vi "DecodeSymbols.vi"(10 "InputValid":bool, 11 "Symbol":T1=enum."Marker") -> (2 "Output Valid":bool, 3 "WWVB":u64 format="%.0x")   [LabVIEW 2019]
uses:
  TypeDefs/TimeSymbol.ctl
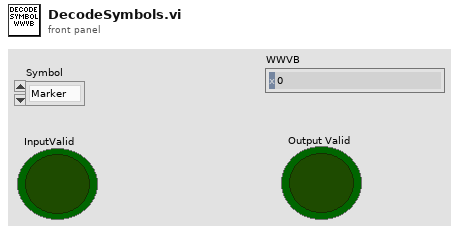
[diagram p1: front panel]
types:
  T1 = typedef "TimeSymbol.ctl" = enum16{"0", "1", "Marker", "Invalid"}
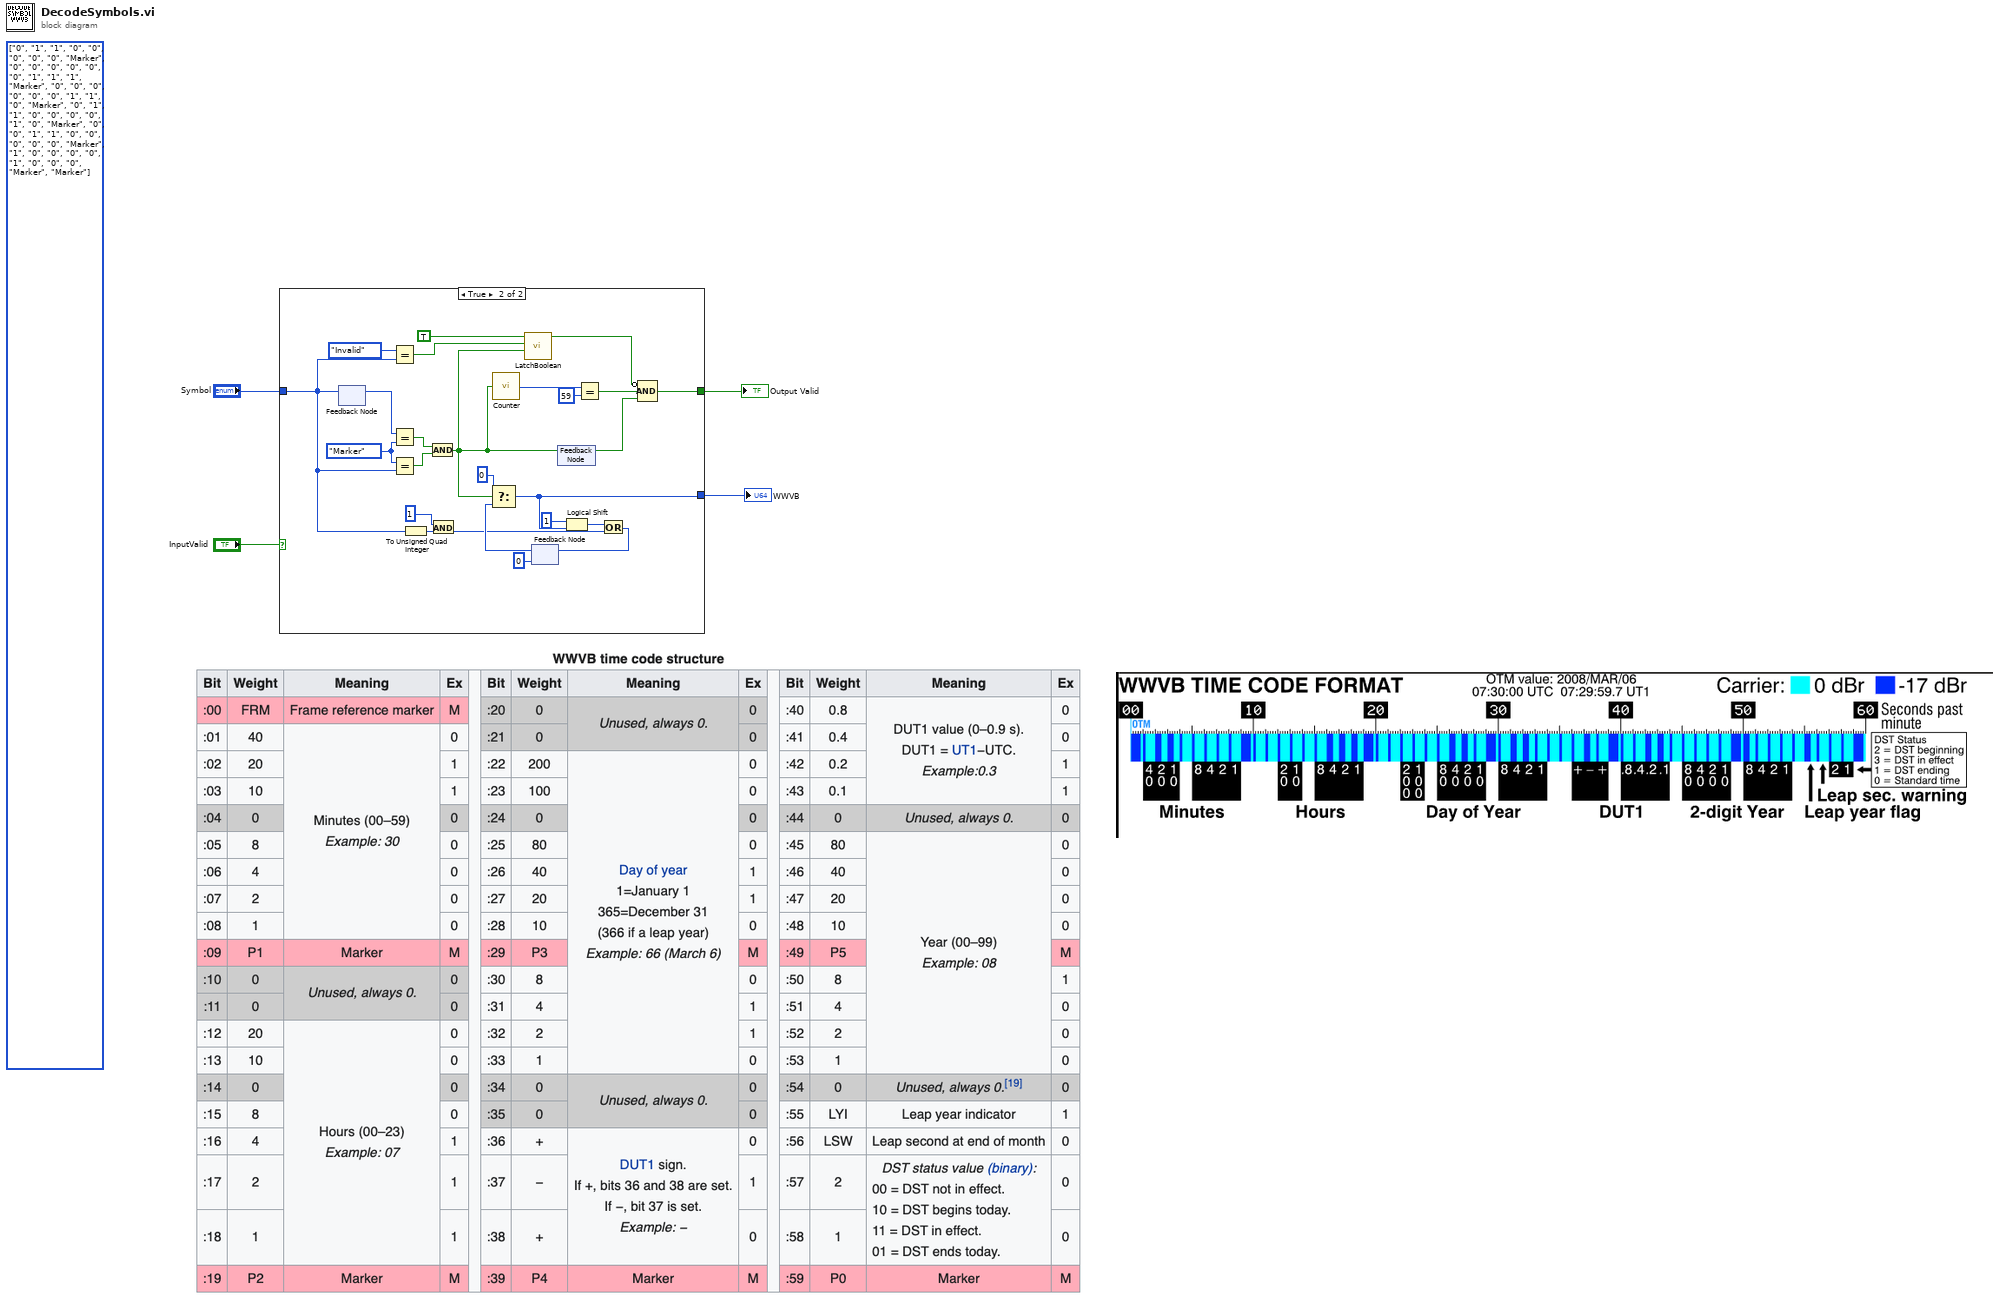
[diagram p0: block diagram]
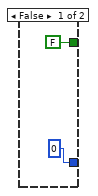
[diagram p2: hidden frame]
diagram:
  (unwired) T1[] [enum."0", enum."1", enum."1", enum."0", enum."0", enum."0", enum."0", enum."0", enum."Marker", enum."0", enum."0", enum."0", enum."0", enum."0", enum."0", enum."1", enum."1", enum."1", enum."Marker", enum."0", enum."0", enum."0", enum."0", enum."0", enum."0", enum."1", enum."1", enum."0", enum."Marker", enum."0", enum."1", enum."1", enum."0", enum."0", enum."0", enum."0", enum."1", enum."0", enum."Marker", enum."0", enum."0", enum."1", enum."1", enum."0", enum."0", enum."0", enum."0", enum."0", enum."Marker", enum."1", enum."0", enum."0", enum."0", enum."0", enum."1", enum."0", enum."0", enum."0", enum."Marker", enum."Marker"] items=["0", "1", "Marker", "Invalid"]
  n1 = case shown="True" "InputValid" {
    tunnel: "Symbol" -> [_ w12]
    tunnel: [u64 0 w16] -> w2
    tunnel: [FALSE w15] -> w1
    frame False {
    }
    frame True {
      w29 = TimeSymbol."Marker" ("Symbol")
      n2 = feedback #1() -> (w31:T1)  [unwired: 1 in]
      n3 = feedback-in #1(w12) -> ()
      n4 = Equal?(x=TimeSymbol."Invalid", y=w12) -> (x = y?=w9:bool)
      n5 = Equal?(x=w31, y=w29) -> (x = y?=w30:bool)
      n6 = Equal?(x=w29, y=w12) -> (x = y?=w28:bool)
      n7 = To Unsigned Quad Integer(1:w12) -> (0:w25:u64)
      n8 = And(x=w30, y=w28) -> (x .and. y?=w10:bool)
      n9 = And(x=u64 1, y=w25) -> (x .and. y?=w22:u64)
      n10 = call "Counter.vi"("Reset"=w10) -> ("Count"=w18:u8)
      n11 = call "LatchBoolean.vi"("Reset"=w10, "Set"=w9, "D"=TRUE ("t")) -> ("Q"=w7:bool)  [unwired: 8 in]
      n12 = feedback #2(u64 0) -> (w23:u64)
      n13 = Select(t=u64 0, s=w10, f=w23) -> (s? t:f=w16:u64)
      n14 = feedback-in #3(w10) -> ()
      n15 = feedback #3() -> (w13:bool)  [unwired: 1 in]
      n16 = Logical Shift(y=i16 1, x=w16) -> (x << y=w19:u64)
      n17 = Equal?(x=w18, y=u8 59) -> (x = y?=w14:bool)
      n18 = Or(x=w19, y=w22) -> (x .or. y?=w24:u64)
      n19 = feedback-in #2(w24) -> ()
      n20 = Compound Arithmetic op=AND(invert w7, w14, w13) -> (w15:bool)
    }
  }
  "WWVB" <- w2
  "Output Valid" <- w1
